vi "master10.vi"() -> ()   [LabVIEW 2013]
uses:
  channel.xctl
panel:
  in  "channel 2":dbl(xcontrol)
  in  "channel 1":dbl(xcontrol)
  in  "Numeric 35":i32=1 min=1 step=1
  in  "Numeric 34":i32=1 min=1 step=1
  in  "Numeric 33":i32=1 min=1 step=1
  in  "Numeric 32":i32=1 min=1 step=1
  in  "Numeric 31":i32=1 min=1 step=1
  in  "Numeric 30":i32=1 min=1 step=1
  in  "Numeric 29":i32=1 min=1 step=1
  in  "Numeric 28":i32=1 min=1 step=1
  in  "Numeric 27":i32=1 min=1 step=1
  in  "Numeric 26":dbl
  in  "Numeric 25":dbl
  in  "Numeric 24":dbl
  in  "Numeric 23":dbl
  in  "Numeric 22":dbl
  in  "Numeric 21":dbl
  in  "Numeric 20":dbl
  in  "Numeric 19":dbl
  in  "Numeric 18":dbl
  in  "Numeric 17":dbl
  in  "Numeric 16":dbl
  in  "Numeric 15":dbl
  in  "Numeric 14":dbl
  in  "Numeric 13":dbl
  in  "Numeric 12":dbl
  in  "Numeric 11":dbl
  in  "Numeric 10":dbl
  in  "Numeric 9":dbl
  in  "Numeric 8":dbl
  in  "Numeric 7":dbl
  in  "Numeric":dbl
  in  "Numeric 6":dbl
  in  "Numeric 5":dbl
  in  "Numeric 4":dbl
  in  "Numeric 3":dbl
  in  "Numeric 2":dbl
  in  "Numeric":dbl
  in  "Save 3":bool
  in  "Save 2":bool
  in  "Save":bool
  in  "Prog 9":u16(ring) items=["Off", "DC", "Trig", "Train", "Gate"]
  in  "Prog 8":u16(ring) items=["Off", "DC", "Trig", "Train", "Gate"]
  in  "Prog 7":u16(ring) items=["Off", "DC", "Trig", "Train", "Gate"]
  in  "Prog 6":u16(ring) items=["Off", "DC", "Trig", "Train", "Gate"]
  in  "Prog 5":u16(ring) items=["Off", "DC", "Trig", "Train", "Gate"]
  in  "Prog 4":u16(ring) items=["Off", "DC", "Trig", "Train", "Gate"]
  in  "Prog 3":u16(ring) items=["Off", "DC", "Trig", "Train", "Gate"]
  in  "Prog 2":u16(ring) items=["Off", "DC", "Trig", "Train", "Gate"]
  in  "Prog 1":u16(ring) items=["Off", "DC", "Trig", "Train", "Gate"]
  out "Waveform Graph":dbl[](graph)
  out "Conn 1 79":bool
  out "Conn 1 78":bool
  out "Conn 1 77":bool
  out "Conn 1 76":bool
  out "Conn 1 75":bool
  out "Conn 1 74":bool
  out "Conn 1 73":bool
  out "Conn 1 72":bool
  out "Conn 1 71":bool
  out "Conn 1 69":bool
  out "Conn 1 68":bool
  out "Conn 1 67":bool
  out "Conn 1 66":bool
  out "Conn 1 65":bool
  out "Conn 1 64":bool
  out "Conn 1 63":bool
  out "Conn 1 62":bool
  out "Conn 1 61":bool
  out "Conn 1 59":bool
  out "Conn 1 58":bool
  out "Conn 1 57":bool
  out "Conn 1 56":bool
  out "Conn 1 55":bool
  out "Conn 1 54":bool
  out "Conn 1 53":bool
  out "Conn 1 52":bool
  out "Conn 1 51":bool
  out "Conn 1 49":bool
  out "Conn 1 48":bool
  out "Conn 1 47":bool
  out "Conn 1 46":bool
  out "Conn 1 45":bool
  out "Conn 1 44":bool
  out "Conn 1 43":bool
  out "Conn 1 42":bool
  out "Conn 1 41":bool
  out "Conn 1 39":bool
  out "Conn 1 38":bool
  out "Conn 1 37":bool
  out "Conn 1 36":bool
  out "Conn 1 35":bool
  out "Conn 1 34":bool
  out "Conn 1 33":bool
  out "Conn 1 32":bool
  out "Conn 1 31":bool
  out "Conn 1 30":bool
  out "Conn 1 29":bool
  out "Conn 1 28":bool
  out "Conn 1 27":bool
  out "Conn 1 26":bool
  out "Conn 1 25":bool
  out "Conn 1 24":bool
  out "Conn 1 23":bool
  out "Conn 1 21":bool
  out "Conn 1 20":bool
  out "Conn 1 19":bool
  out "Conn 1 18":bool
  out "Conn 1 17":bool
  out "Conn 1 16":bool
  out "Conn 1 14":bool
  out "Conn 1 13":bool
  out "Conn 1 12":bool
  out "Conn 1 11":bool
  out "Conn 1 10":bool
  out "Conn 1 9":bool
  out "Conn 1 8":bool
  out "Conn 1 7":bool
  out "Conn 1 6":bool
  out "Conn 1 4":bool
  out "Conn 1 3":bool
  out "Conn 1 3":bool
  out "Conn 1 2":bool
  # "Delay"
  # "Duration"
  # "Interval"
  # "N"
  # "Analog"
  # "Analog Randomiize\nSequence\nJittered Delay"
  # "Connection Origin"
  # "1"
  # "1"
  # "2"
  # "3"
  # "4"
  # "5"
  # "6"
  # "7"
  # "8"
  # "9"
  # "Connection Target"
  # "2"
  # "1"
  # "2"
  # "3"
  # "3"
  # "4"
  # "4"
  # "5"
  # "5"
  # "6"
  # "6"
  # "7"
  # "8"
  # "7"
  # "9"
  # "8"
  # "9"
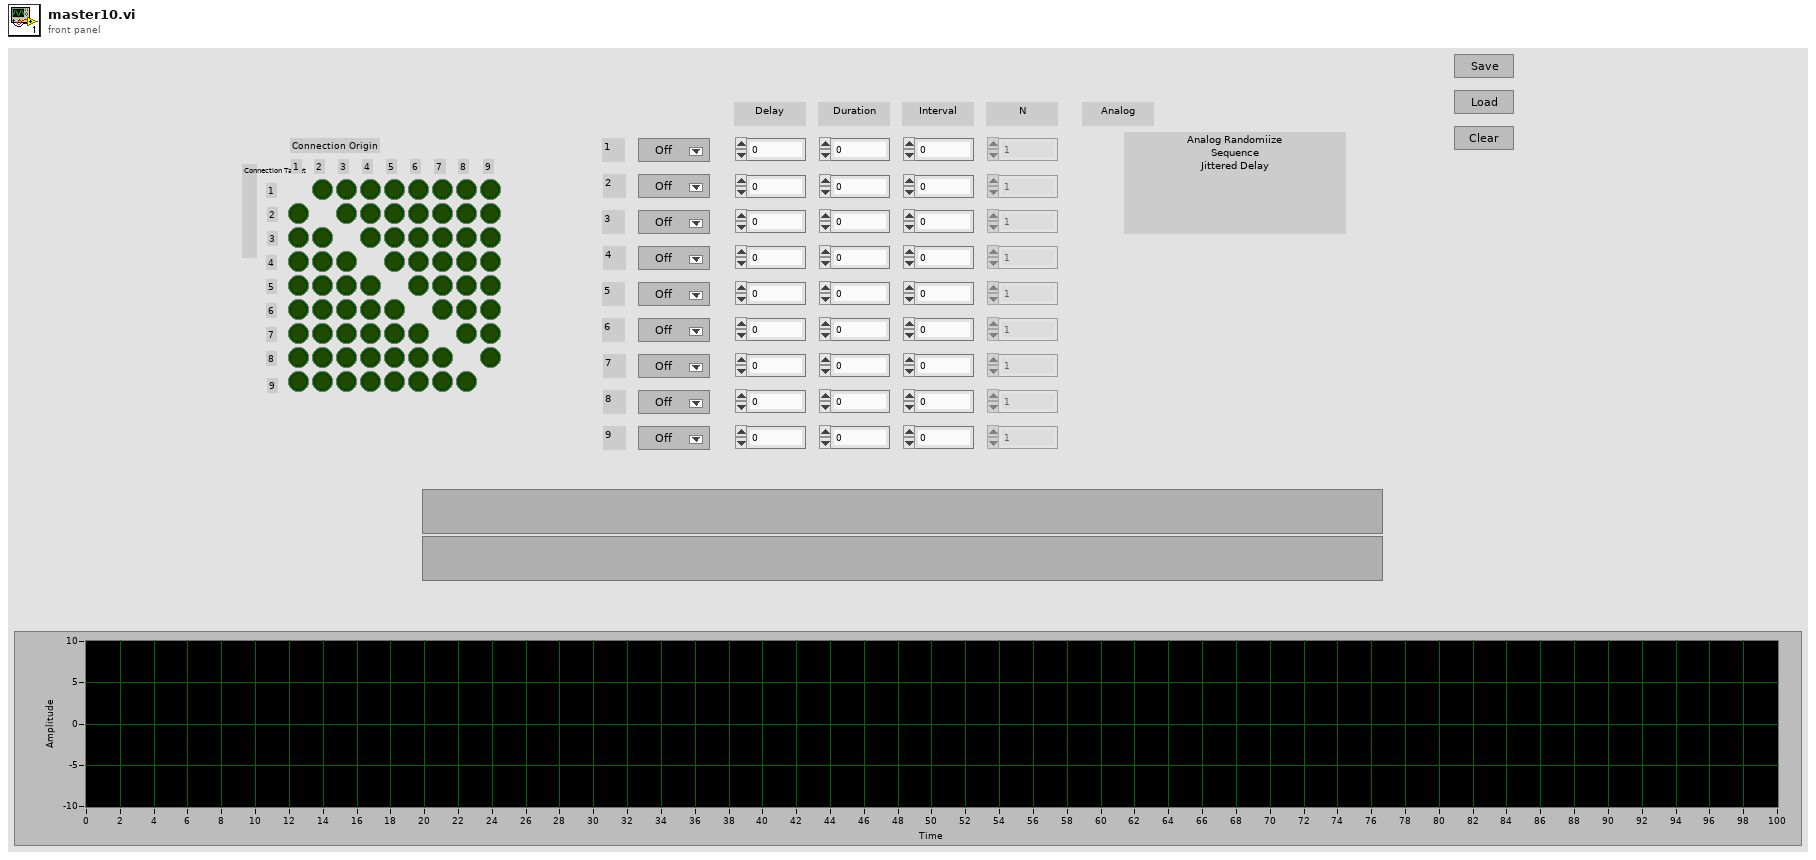
[diagram p1: front panel]
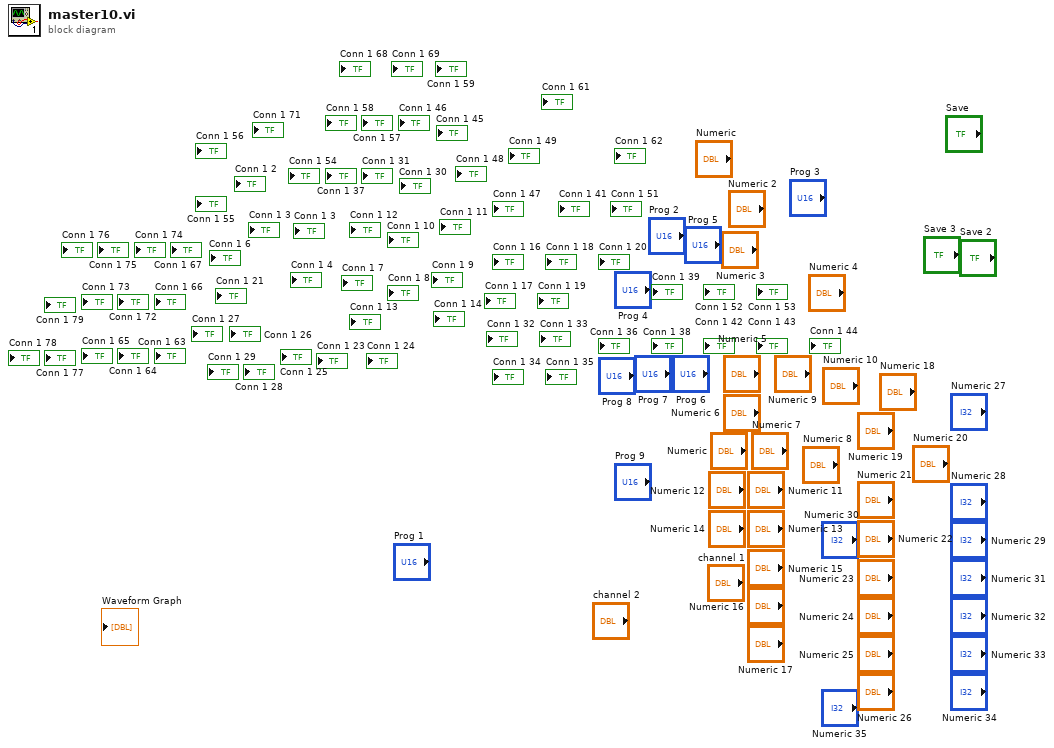
[diagram p0: block diagram]
diagram:
